vi "103_Execute_Build_Specs_G-CLI.vi"() -> ()   [LabVIEW 2023]
doc: "Execute Build Specs G-CLI.vi\n----------------------------------------------\nThis VI is used to build the lvlibp from the build specifications.\n\nInputs:\n---------------------\n\n\nOutputs:\n---------------------\n\n\n----------------------------------------------\n1/27/2021 nina\nZühlke Engineering AG\nCH-8952 Schlieren\nwww.zuehlke.com"
uses:
  <vilib>/AppBuilder/AB_API_Simple/Get Build Specification Version (path).vi
  <vilib>/Wiresmith Technology/G CLI/CLI Class/CLI.lvclass
  <vilib>/AppBuilder/AB_API_Simple/NI_App_Builder_API.lvlib
panel:
  out "error out":errorcluster
  out "Build Specification Names":string[](array[string])
  # "Locals"
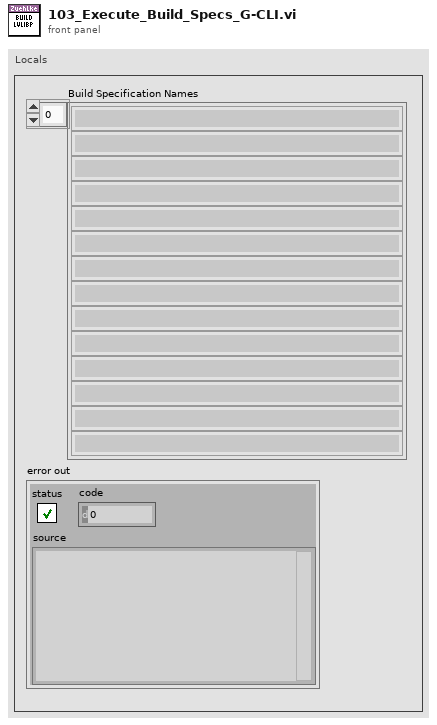
[diagram p1: front panel]
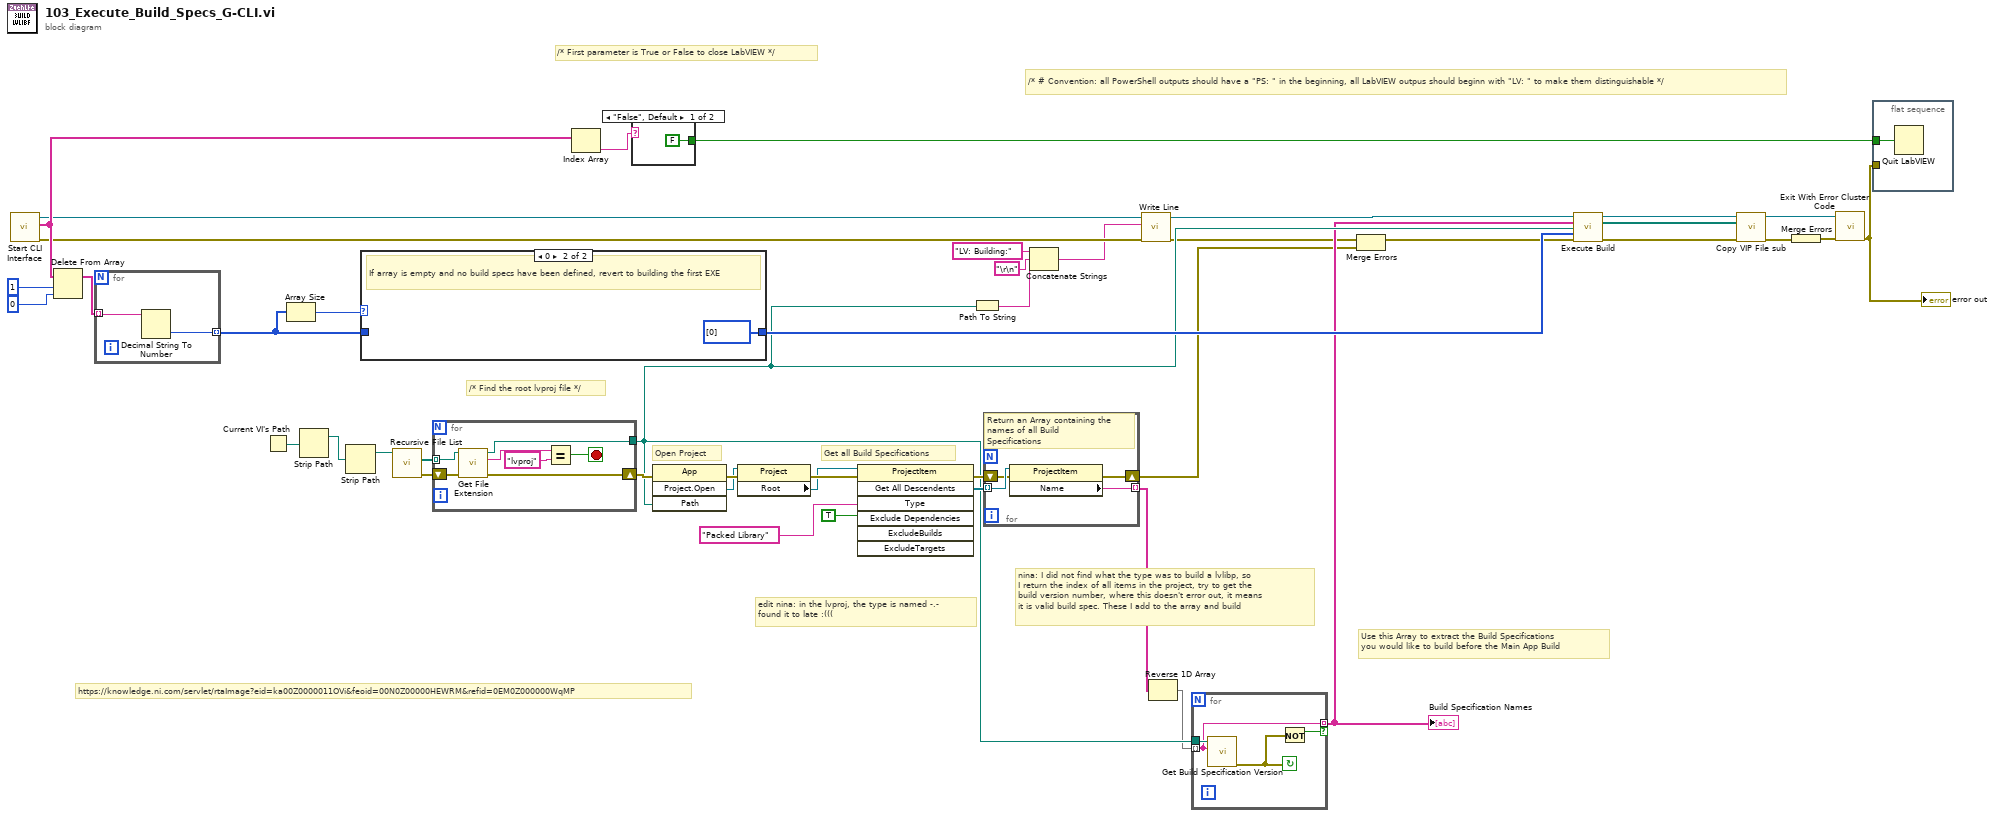
[diagram p0: block diagram]
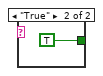
[diagram p2: hidden frame]
diagram:
  # "/* # Convention: all PowerShell outputs should have a \"PS: \" in the beginning, all LabVIEW outpus should beginn with \"LV: \" to make them distinguishable */"
  # "edit nina: in the lvproj, the type is named -.-\nfound it to late :((("
  # "nina: I did not find what the type was to build a lvlibp, so\nI return the index of all items in the project, try to get the \nbuild version number, where this doesn't error out, it means\nit is valid build spec. These I add to the array and build"
  # "/* First parameter is True or False to close LabVIEW */"
  # "Use this Array to extract the Build Specifications \nyou would like to build before the Main App Build"
  # "Get all Build Specifications"
  # "Open Project"
  # "https://knowledge.ni.com/servlet/rtaImage?eid=ka00Z0000011OVi&feoid=00N0Z00000HEWRM&refid=0EM0Z000000WqMP"
  # "/* Find the root lvproj file */"
  n1 = call <vilib>:"Start CLI Interface.vi"() -> ("error out"=w20:errorcluster, "Custom Parameters"=w26:string[], "CLI out"=w22:refnum<class "CLI.lvclass">)  [unwired: 8 in, 1 out]
  n2 = Delete From Array(array=w26, length=1, index=0) -> (array with subset deleted=w23:string[])  [unwired: 1 out]
  n3 = for {
    tunnel: w23 -> [w46] mode=indexing
    tunnel: [w45] -> w30 mode=indexing
    n4 = Decimal String To Number(string=w46) -> (number=w45:i32)  [unwired: 2 in, 1 out]
  }
  n5 = Current VI's Path() -> (path=w44:path)
  n6 = Array Size(array=w30) -> (size(s)=w31:i32)
  n7 = Strip Path(path=w44) -> (stripped path=w41:path)  [unwired: 1 out]
  n8 = Strip Path(path=w41) -> (stripped path=w16:path)  [unwired: 1 out]
  n9 = case shown="0" w31 {
    tunnel: w30 -> [w47 _]
    tunnel: [w47 i32[] [0]] -> w29
    frame Default {
    }
    frame 0 {
      # "If array is empty and no build specs have been defined, revert to building the first EXE"
    }
  }
  n10 = call <vilib>:"Recursive File List.vi"("Folder Path"=w16) -> ("error out"=w42:errorcluster, "All Files in Dir"=w43:path[])  [unwired: 6 in, 3 out]
  n11 = for {
    tunnel: w43 -> [w55] mode=indexing
    tunnel: [w51] -> w15
    shift-right: [w49] -> w33
    shift-left: w42 -> [w50]
    stop <- w52 stop-if-true
    n12 = call <vilib>:"Get File Extension.vi"("error in (no error)"=w50, "file"=w55) -> ("error out"=w49:errorcluster, "lowercase file extension"=w54:string, "dup file"=w51:path)  [unwired: 5 in, 2 out]
    n13 = Equal?(x=w54, y="lvproj") -> (x = y?=w52:bool)
  }
  n14 = Index Array(array=w26) -> (element=w28:string)  [unwired: 1 in]
  n15 = case shown="\"False\", Default" w28 {
    tunnel: [FALSE TRUE] -> w27
    frame "False", Default {
    }
    frame "True" {
    }
  }
  n16 = invoke class="App" method="Project.Open"(error in=w33, "Path"=w15) -> (error out=w37:errorcluster, "Project:Open"=w36:refnum<vi>)  [unwired: 2 in, 2 out]
  n17 = property class="Project"(reference=w36, error in=w37) -> (error out=w39:errorcluster, "Root"=w38:refnum<vi>)  [unwired: 1 out]
  n18 = invoke class="ProjectItem" method="Get All Descendents"(reference=w38, error in=w39, "Type"="Packed Library", "Exclude Dependencies"=TRUE ("ExcludeDependencies")) -> (error out=w34:errorcluster, "All Descendents"=w35:refnum<vi>[])  [unwired: 3 in, 5 out]
  n19 = Path To String(path=w15) -> (string=w17:string)
  n20 = for {
    tunnel: w35 -> [w61] mode=indexing
    tunnel: [w60] -> w14 mode=indexing
    shift-right: [w58] -> w3
    shift-left: w34 -> [w59]
    # "Return an Array containing the names of all Build Specifications"
    n21 = property class="ProjectItem"(reference=w61, error in=w59) -> (error out=w58:errorcluster, "Name"=w60:string)  [unwired: 1 out]
  }
  n22 = Concatenate Strings("LV: Building:" ("string"), "\r\n", w17) -> (w1:string)
  n23 = call <vilib>:"Write Line.vi"("error in (no error)"=w20, "Text to Write"=w1, "CLI in"=w22) -> ("error out"=w6:errorcluster, "CLI out"=w21:refnum<class "CLI.lvclass">)  [unwired: 7 in]
  n24 = Reverse 1D Array(array=w14) -> (reversed array=w13:string[])
  n25 = for {
    tunnel: w15 -> [w65]
    tunnel: w13 -> [w64] mode=indexing
    tunnel: [w64] -> w12 mode=indexing if=w63
    stop <- w62 continue-if-true
    n26 = call-poly <vilib>:"Get Build Specification Version.vi"("Name of build specification"=w64, "Path to project"=w65) -> ("error out"=w62:errorcluster)  [unwired: 8 in, 1 out]
    n27 = Not(x=w62) -> (.not. x?=w63:bool)
  }
  "Build Specification Names" <- w12
  n28 = Merge Errors(w6, w3) -> (w4:errorcluster)
  n29 = call "Execute Build.vi"("CLI in"=w21, "All Build Specs"=w12, "Proj Path"=w15, "Specs to be built"=w29, "error in (no error)"=w4) -> ("CLI out"=w9:refnum<class "CLI.lvclass">, "Created Files"=w10:path[], "error out"=w5:errorcluster)  [unwired: 8 in]
  n30 = call "Copy VIP File sub.vi"("CLI in"=w9, "Array of created files"=w10, "error in (no error)"=w5) -> ("CLI out"=w8:refnum<class "CLI.lvclass">, "error out"=w7:errorcluster)  [unwired: 11 in]
  n31 = Merge Errors(w7) -> (w32:errorcluster)
  n32 = call <vilib>:"Exit With Error Cluster Code.vi"("error in (no error)"=w32, "CLI in"=w8) -> ("error out"=w2:errorcluster)  [unwired: 9 in]
  "error out" <- w2
  n33 = flat-sequence {
    tunnel: w27 -> [w66]
    tunnel: w2 -> [_]
    frame #0 {
      n34 = Quit LabVIEW(quit? (T)=w66) -> ()
    }
  }
